vi "Build Speed Frequency XY Graph Data.vi"(8 "maximum freq":dbl, 9 "maximum speed":dbl, 10 "min freq":dbl) -> (3 "XY data":cluster{dbl, dbl}[](array[cluster]))   [LabVIEW 2013, in "Engine Simulation Toolkit System Explorer.lvlib"]
uses:
  Engine Simulation Toolkit System Explorer.lvlib
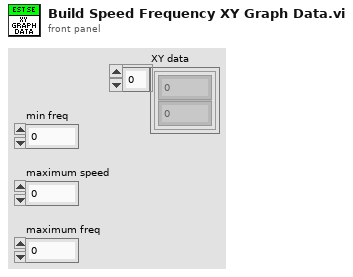
[diagram p1: front panel]
types:
  T1 = cluster{"maximum speed":dbl, "maximum freq":dbl}[]
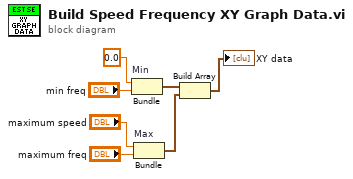
[diagram p0: block diagram]
diagram:
  n1 = Bundle "Min"("min speed"=0.0, "min freq"="min freq") -> (w6:cluster{"min speed":dbl, "min freq":dbl})  [unwired: 1 in]
  n2 = Bundle "Max"("maximum speed"="maximum speed", "maximum freq"="maximum freq") -> (w7:cluster{"maximum speed":dbl, "maximum freq":dbl})  [unwired: 1 in]
  n3 = Build Array(w6, w7) -> (→"XY data":T1)
